vi "Trigger_measurement.vi"(8 "refnum":refnum<file>, 9 "Number of Pulses":i32, 10 "position":string, 11 "VISA resource name":refnum<visa-resource-name>="COM4") -> (0 "refnum out":refnum<file>, 1 "charge(C)":dbl, 2 "Response":string, 3 "VISA resource name out":refnum<visa-resource-name>)   [LabVIEW 2024]
doc: "This example performs writes and reads on a serial port, as directed by the user. You can press the Write and Read buttons, and change the Read Count, while the example is running.\n\nThe parameters set for the serial port must match the parameters of the connected instrument or device. In this example, the Read Count parameter specifies the number of bytes that the serial port reads. If there were more bytes at the port than the specified number, those bytes would not be read. If there were less bytes at the port than the specified number, you would receive a timeout error.\n\nThis example expands upon the flow control options for XON and XOFF, allowing the user to choose those control characters. Also, the user can enable or disable a termination character. Some devices require a termination character in order to identify the end of command strings. Some devices send a termination character to signify the end of data to be read. This example shows how you can end the Read operation once a termination character is detected in the buffer and/or append a termination character at the end of the Write data."
uses:
  support/Serial - XON-XOFF Characters.ctl
  support/Serial - ASCII Characters.ctl
  support/Serial - Settings.ctl
  <vilib>/Instr/_visa.llb/VISA Configure Serial Port (Instr).vi
panel:
  in  "Read Count":u32=1000
  out "return count":u32=10
  # "Overview: Demonstrates the use of the VISA functions to write commands to and read responses from a serial instrument continuously in a loop.\nRequirements: NI-VISA Driver\nInstructions:\n1. Run the VI.\n2. Specify a Command and click the Write button.\n3. Read a Response by clicking the Read button.\n4. Click Stop to stop the VI."
  # "Multi-Commands can be given in one command if seperated by semicolons"
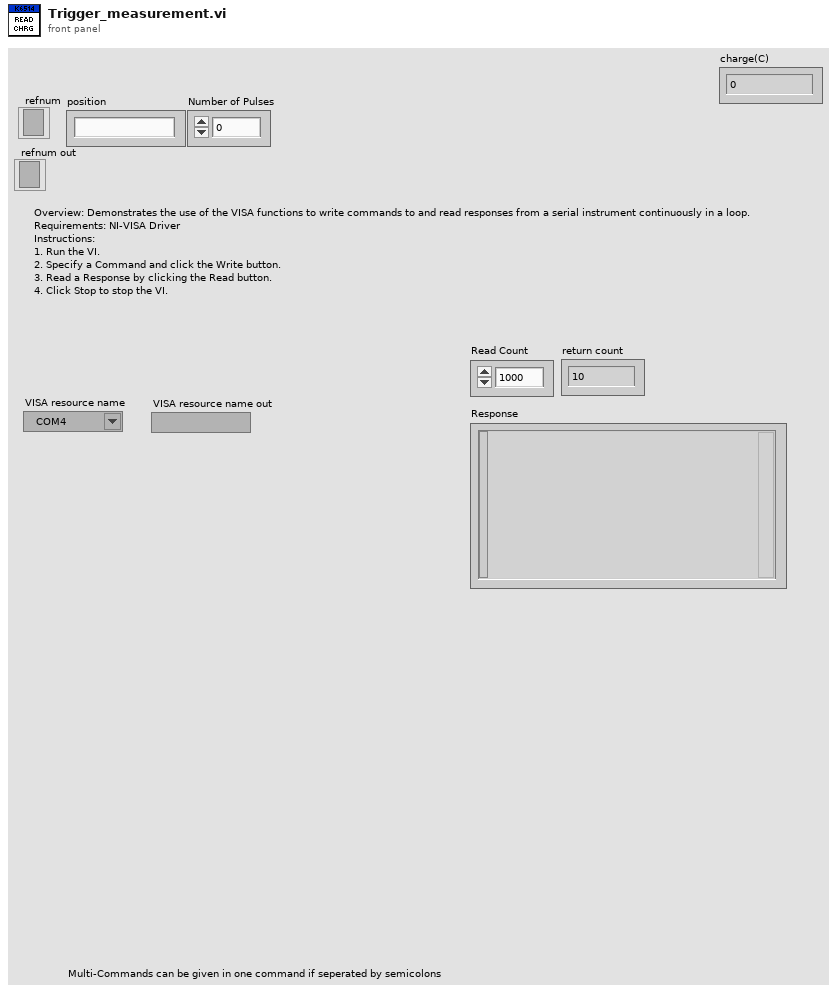
[diagram p1: front panel]
types:
  T1 = typedef "Serial - Settings.ctl" = cluster{"baud rate":u32, "data bits":u16, "parity":enum16{"None", "Odd", "Even", "Mark", "Space"}, "stop bits":u16, "flow control":u16}
  T2 = typedef "Serial - XON-XOFF Characters.ctl" = cluster{"XON":T3, "XOFF":T3}
  T3 = typedef "Serial - ASCII Characters.ctl" = enum16{"NUL", "SOH", "STX", "ETX", "EOT", "ENQ", "ACK", "BEL", "BS", "HT", "LF", "VT", "FF", "CR", "SO", "SI", "DLE", "DC1", "DC2", "DC3", "DC4", "NAK", "SYN", "ETB", "CAN", "EM", "SUB", "ESC", "FS", "GS", "RS", "US", "SP", "!", "\"", "#", "$", "%", "&", "'", "(", ")", "*", "+", ",", "- (-)", ".", "/", "0", "1", "2", "3", "4", "5", "6", "7", "8", "9", ":", ";", "<", "=", ">", "?", "@", "A", "B", "C", "D", "E", "F", "G", "H", "I", "J", "K", "L", "M", "N", "O", "P", "Q", "R", "S", "T", "U", "V", "W", "X", "Y", "Z", "[", "\\", "]", "^", "_", "`", "a", "b", "c", "d", "e", "f", "g", "h", "i", "j", "k", "l", "m", "n", "o", "p", "q", "r", "s", "t", "u", "v", "w", "x", "y", "z", "{", "|", "}", "~"}
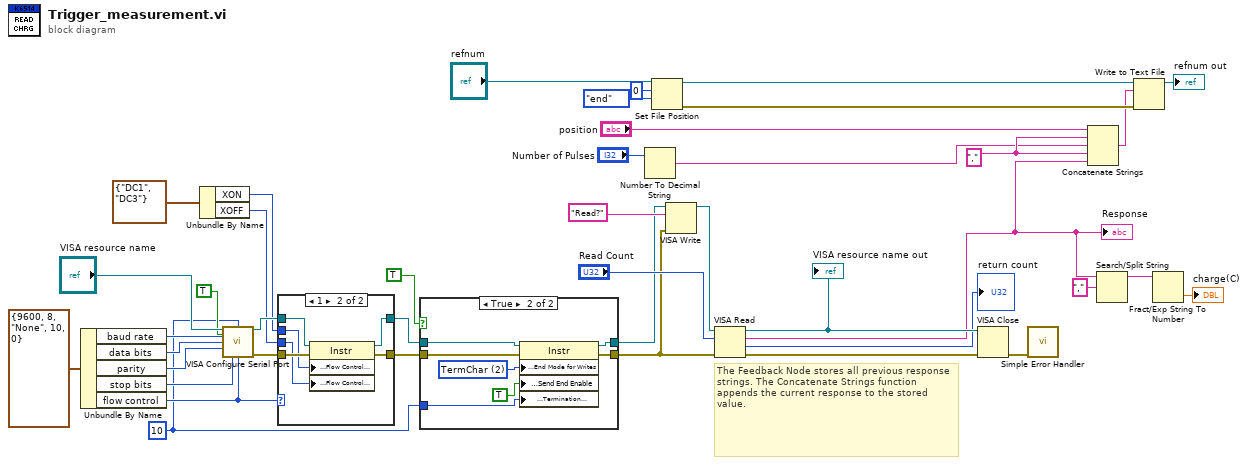
[diagram p0: block diagram]
diagram:
  w9 = "," ("string")
  w25 = u8 10 ("Termination Character")
  # "The Feedback Node stores all previous response strings. The Concatenate Strings function appends the current response to the stored value."
  n1 = Unbundle By Name(T1 {"baud rate"=9600, "data bits"=8, "parity"=enum."None", "stop bits"=10, "flow control"=0} ("Serial Settings")) -> ("baud rate"=w34:u32, "data bits"=w35:u16, "parity"=w36:enum16{"None", "Odd", "Even", "Mark", "Space"}, "stop bits"=w37:u16, "flow control"=w31:u16)
  n2 = Unbundle By Name(T2 {"XON"=enum."DC1", "XOFF"=enum."DC3"} ("XON/XOFF Characters")) -> ("XON"=w30:T3, "XOFF"=w29:T3)
  n3 = call-poly "VISA Configure Serial Port"("VISA resource name"="VISA resource name", "termination char\n(0xA = '\\n' = LF)"=w25, "Enable Termination\nChar (T)"=TRUE ("End Read on Termination Character?"), "baud rate (9600)"=w34, "data bits (8)"=w35, "parity (0:none)"=w36, "stop bits (10: 1 bit)"=w37, "flow control (0:none)"=w31) -> ("VISA resource name out"=w38:refnum<visa-resource-name>, "error out"=w39:errorcluster)  [unwired: 2 in, 4 out]
  n4 = case shown="1" w31 {
    tunnel: [w42 w49] -> w28
    tunnel: [w43 w48] -> w27
    tunnel: w39 -> [w42 w47]
    tunnel: w38 -> [w43 w46]
    tunnel: w30 -> [_ w45]
    tunnel: w29 -> [_ w44]
    frame Default {
    }
    frame 1 {
      n5 = property class="Instr"(reference=w46, error in=w47, "Serial Settings:Flow Control XON Character"=w45, "Serial Settings:Flow Control XOFF Character"=w44) -> (reference out=w48:refnum<visa-resource-name>, error out=w49:errorcluster)
    }
  }
  n6 = case shown="True" TRUE ("End Write on Termination Character?") {
    tunnel: w27 -> [w50 w58]
    tunnel: w28 -> [w51 w57]
    tunnel: [w50 w56] -> w18
    tunnel: [w51 w55] -> w17
    tunnel: w25 -> [_ w53]
    frame False {
    }
    frame True {
      w54 = u16 2 items=["None", "LastBit", "TermChar", "Break"] ("Serial Settings:Serial End Mode for Writes")
      n7 = property class="Instr"(reference=w58, error in=w57, "Serial Settings:End Mode for Writes"=w54, "Message Based Settings:Send End Enable"=TRUE, "Message Based Settings:Termination Character"=w53) -> (reference out=w56:refnum<visa-resource-name>, error out=w55:errorcluster)
    }
  }
  n8 = Number To Decimal String(number="Number of Pulses") -> (decimal integer string=w6:string)  [unwired: 1 in]
  n9 = Set File Position(offset (in bytes) (0)=i64 0, refnum="refnum", from (0:start)=enum16{"start", "end", "current"}."end") -> (refnum out=w12:refnum<file>, error out=w15:errorcluster)  [unwired: 1 in]
  n10 = VISA Write(VISA resource name=w18, write buffer="Read?" ("String"), error in (no error)=w17) -> (VISA resource name out=w16:refnum<visa-resource-name>)  [unwired: 2 out]
  n11 = VISA Read(VISA resource name=w16, byte count="Read Count", error in (no error)=w17) -> (VISA resource name out=w22:refnum<visa-resource-name>, read buffer=w4:string, return count=→"return count":u32, error out=w23:errorcluster)
  "Response" <- w4
  "VISA resource name out" <- w22
  n12 = VISA Close(VISA resource name=w22, error in (no error)=w23) -> (error out=w24:errorcluster)
  n13 = call <vilib>:"Simple Error Handler.vi"("error in (no error)"=w24) -> ()  [unwired: 1 in, 8 out]
  n14 = Concatenate Strings("position", w9, w6, w9, w4) -> (w8:string)
  n15 = Search/Split String(string=w4, search string/char (-)=",") -> (substring before match=w2:string)  [unwired: 1 in, 2 out]
  n16 = Write to Text File(file (use dialog)=w12, text=w8, error in=w15) -> (refnum out=→"refnum out":refnum<file>)  [unwired: 1 in, 2 out]
  n17 = Fract/Exp String To Number(string=w2) -> (number=→"charge(C)":dbl)  [unwired: 3 in, 1 out]
